vi "Get Error Codes File Properties.vi"(8 "error in (no error)":errorcluster, 11 "error list <owner> in":variant) -> (0 "error out":errorcluster, 1 "found?":bool, 2 "properties":T1, 3 "error list <owner> out":variant)   [LabVIEW 2017]
uses:
  Error Code File Properties.ctl
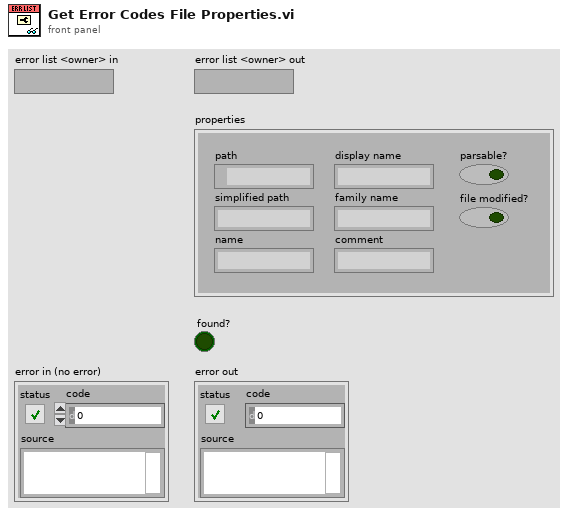
[diagram p1: front panel]
types:
  T1 = typedef "Error Code File Properties.ctl" = cluster{"path":path, "simplified path":string, "name":string, "display name":string, "family name":string, "comment":string, "parsable?":bool, "file modified?":bool}
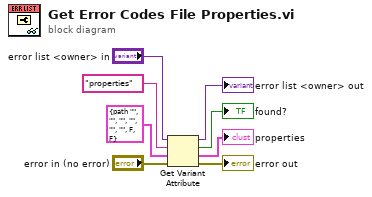
[diagram p0: block diagram]
diagram:
  n1 = Get Variant Attribute(Variant="error list <owner> in", name="properties", default value (empty Variant)=T1 {"path"=path "", "simplified path"="", "name"="", "display name"="", "family name"="", "comment"="", "parsable?"=FALSE, "file modified?"=FALSE} ("error code file"), error in="error in (no error)") -> (duplicate Variant=→"error list <owner> out":variant, found=→"found?":bool, value=→"properties":T1, error out=→"error out":errorcluster)
